vi "ep_Get Sideband Window Parameters.vi"(7 "demodulated? (F)":bool, 8 "error in (no error)":errorcluster, 9 "search +/- percentage":dbl, 10 "search information":T1, 11 "k":i32=1) -> (0 "error out":errorcluster, 2 "sideband window":T2={"sideband frequency"=0.0, "number of half window length "=1, "fbrb in range? (F)"=FALSE})   [LabVIEW 2014, in "NI_EP_Motor Monitoring.lvlib"]
uses:
  <vilib>/addons/Electrical Power/Motor Monitoring/NI_EP_Motor Monitoring.lvlib
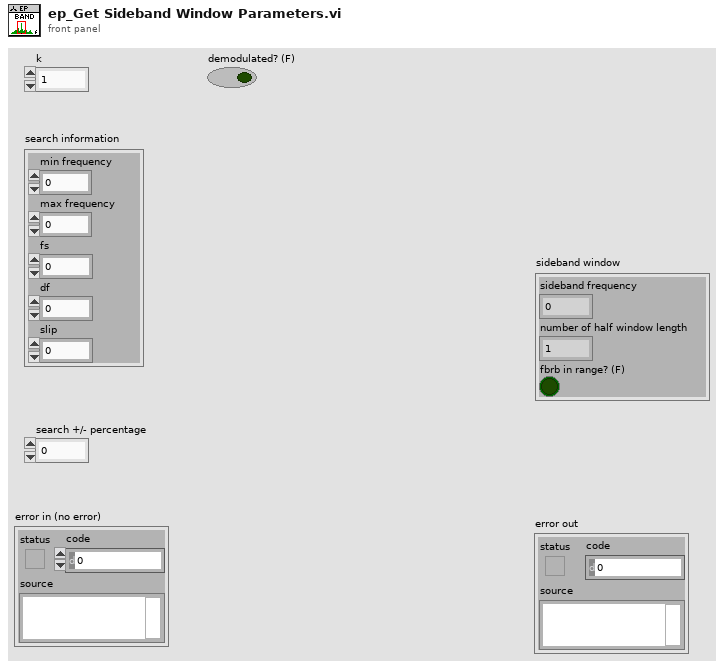
[diagram p1: front panel]
types:
  T1 = cluster{"min frequency":dbl, "max frequency":dbl, "fs":dbl, "df":dbl, "slip":dbl}
  T2 = cluster{"sideband frequency":dbl, "number of half window length ":u8, "fbrb in range? (F)":bool}
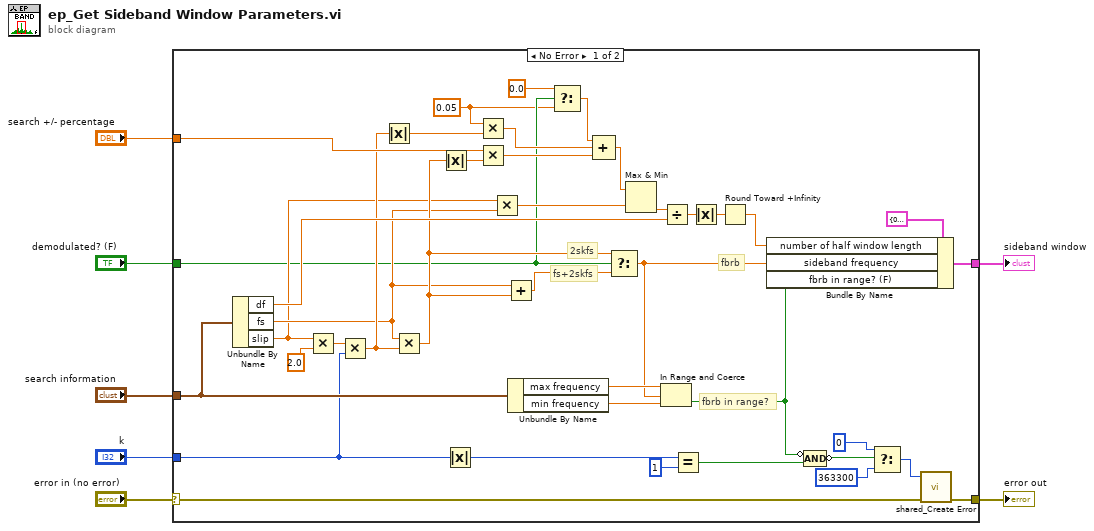
[diagram p0: block diagram]
diagram:
  n1 = case shown="No Error" "error in (no error)" {
    selector: "error in (no error)" -> [w45 w48]
    tunnel: "k" -> [w22 _]
    tunnel: [w34 w48] -> w4
    tunnel: "demodulated? (F)" -> [w11 _]
    tunnel: "search information" -> [w36 _]
    tunnel: [w39 _] -> w1
    tunnel: "search +/- percentage" -> [w29 _]
    frame No Error {
      w8 = 0.05 ("y")
      # "fs+2skfs"
      # "2skfs"
      # "fbrb"
      # "fbrb in range?"
      n2 = Unbundle By Name(w36) -> ("df"=w30:dbl, "fs"=w14:dbl, "slip"=w13:dbl)
      n3 = Multiply(x=w13, y=2.0 ("x")) -> (x*y=w31:dbl)
      n4 = Multiply(x=w31, y=w22) -> (x*y=w21:dbl)
      n5 = Absolute Value(x=w21) -> (abs(x)=w20:dbl)
      n6 = Multiply(x=w14, y=w21) -> (x*y=w17:dbl)
      n7 = Absolute Value(x=w17) -> (abs(x)=w18:dbl)
      n8 = Absolute Value(x=w22) -> (abs(x)=w40:i32)
      n9 = Multiply(x=w8, y=w20) -> (x*y=w19:dbl)
      n10 = Multiply(x=w29, y=w18) -> (x*y=w16:dbl)
      n11 = Multiply(x=w13, y=w14) -> (x*y=w15:dbl)
      n12 = Add(x=w14, y=w17) -> (x+y=w25:dbl)
      n13 = Unbundle By Name(w36) -> ("max frequency"=w43:dbl, "min frequency"=w28:dbl)
      n14 = Select(t=0.0 ("y"), s=w11, f=w8) -> (s? t:f=w10:dbl)
      n15 = Compound Arithmetic op=ADD(w10, w19, w16) -> (w12:dbl)
      n16 = Select(t=w17, s=w11, f=w25) -> (s? t:f=w26:dbl)
      n17 = Max & Min(x=w12, y=w15) -> (min(x,y)=w32:dbl)  [unwired: 1 out]
      n18 = In Range and Coerce(upper limit=w43, x=w26, lower limit=w28) -> (In Range?=w33:bool)  [unwired: 1 out]
      n19 = Divide(x=w32, y=w30) -> (x/y=w38:dbl)
      n20 = Equal?(x=w40, y=1) -> (x = y?=w41:bool)
      n21 = Absolute Value(x=w38) -> (abs(x)=w37:dbl)
      n22 = Round Toward +Infinity(x=w37) -> (ceil(x): smallest int >= x=w27:dbl)
      n23 = Bundle By Name(cluster=T2 {"sideband frequency"=0.0, "number of half window length "=1, "fbrb in range? (F)"=FALSE} ("sideband window"), "number of half window length"=w27, "sideband frequency"=w26, "fbrb in range? (F)"=w33) -> (w39:T2)
      n24 = Compound Arithmetic op=AND(invert w33, w41) -> (invert w35:bool)
      n25 = Select(t=0 ("error code (0)"), s=w35, f=363300 ("error code (0)")) -> (s? t:f=w46:i32)
      n26 = call <vilib>:"shared_Create Error.vi"("error in (no error)"=w45, "error code (0)"=w46) -> ("error out"=w34:errorcluster)  [unwired: 9 in]
    }
    frame Error {
    }
  }
  "sideband window" <- w1
  "error out" <- w4
